vi "删除1D数组元素(VI-REF).vi"(8 "error in (no error)":errorcluster caption="错误输入（无错误）", 10 "索引":i32[](array[numeric]), 11 "输入数组":refnum<vi>[](array[refnum])) -> (0 "error out":errorcluster caption="错误输出", 2 "已删除元素":refnum<vi>[](array[refnum]), 3 "剩余元素":refnum<vi>[](array[refnum]))   [LabVIEW 2012]
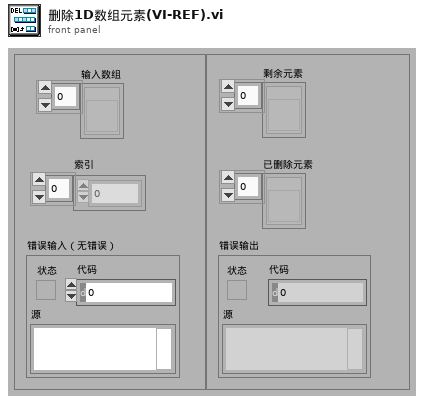
[diagram p1: front panel]
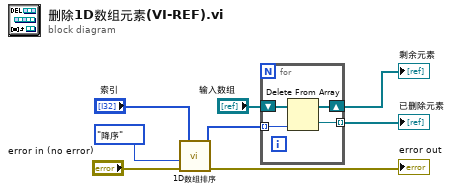
[diagram p0: block diagram]
diagram:
  n1 = call-poly "1D数组排序.vi"("error in (no error)"="error in (no error)", "升降序"=enum16{"升序", "降序"}."降序", "输入数组"="索引") -> ("error out"=→"error out":errorcluster, "排序后数组"=w4:i32[])  [unwired: 6 in, 1 out]
  n2 = for {
    shift-right: [w11] -> w3
    shift-left: "输入数组" -> [w12]
    tunnel: w4 -> [w10] mode=indexing
    tunnel: [w9] -> w1 mode=indexing
    n3 = Delete From Array(array=w12, index=w10) -> (deleted portion=w9:refnum<vi>, array with subset deleted=w11:refnum<vi>[])  [unwired: 1 in]
  }
  "剩余元素" <- w3
  "已删除元素" <- w1
